vi "Triaxial Aquisition.vi"() -> ()   [LabVIEW 2017]
uses:
  <vilib>/UPVI/lvhdf5/dataset.llb/LVH5D Operation.ctl
  <vilib>/Utility/miscctls.llb/LVRectTypeDef.ctl
  <vilib>/UPVI/lvhdf5/attribute.llb/LVH5A Operation.ctl
  <vilib>/UPVI/lvhdf5/group.llb/H5G_obj_t.ctl
  <vilib>/UPVI/lvhdf5/file.llb/LVH5F Operation.ctl
  <vilib>/UPVI/lvhdf5/identifier.llb/Not an HDF5 Refnum Constant.vi
  <vilib>/UPVI/lvhdf5/common.llb/To HDF5 Ref.vi
  <vilib>/express/express analysis/Spectral/Block/exnSpectralBlock spectral measurements power poly.vi
  <vilib>/express/express analysis/Spectral/Block/exnSpectralBlock spectral measurements power DDT.vi
  <vilib>/UPVI/lvhdf5/file.llb/OpenCreateReplace HDF5 File.vi
  <vilib>/UPVI/lvhdf5/utility.llb/Select HDF5 Dialog.vi
  <vilib>/UPVI/lvhdf5/utility.llb/Select HDF5 Dialog (File and Object).vi
  <vilib>/UPVI/lvhdf5/dataset.llb/Simple H5Dwrite (Variant).vi
  <vilib>/UPVI/lvhdf5/attribute.llb/Write Multiple Attributes.vi
  <vilib>/UPVI/lvhdf5/dataset.llb/H5Dclose.vi
  <vilib>/express/express analysis/Spectral/XNode/ExpressSpectralMeasurementsBlockNode.xnode
  <vilib>/UPVI/lvhdf5/dataset.llb/Write Dataset with Attributes.xnode
  <vilib>/UPVI/lvhdf5/library.llb/HDF5 Ref.ctl
  <vilib>/Utility/error.llb/Error Cluster From Error Code.vi
  <vilib>/UPVI/lvhdf5/dataset.llb/OpenCreateReplace Dataset by Element Type.vi
  <vilib>/UPVI/lvhdf5/dataspace.llb/H5Sselect_hyperslab.vi
  <vilib>/UPVI/lvhdf5/dataset.llb/H5Dwrite (Variant).vi
  <vilib>/UPVI/lvhdf5/dataset.llb/H5Dget_space.vi
  <vilib>/UPVI/lvhdf5/attribute.llb/private/LVH5AwriteWDTAttrs.vi
  <vilib>/UPVI/lvhdf5/dataspace.llb/H5Sclose.vi
  <vilib>/UPVI/lvhdf5/utility.llb/Select HDF5 Dialog (Object Only).vi
  <vilib>/Utility/VariantDataType/GetClusterInfo.vi
  <vilib>/Utility/VariantDataType/VariantType.lvlib
  <vilib>/Utility/VariantDataType/GetTypeInfo.vi
  <vilib>/UPVI/lvhdf5/attribute.llb/Cluster to Attribute Array.xnode
panel:
  out "Array":dbl[][](array[numeric])
  out "Z":dynamicdata(graph)
  out "Y":dynamicdata(graph)
  out "X":dynamicdata(graph)
  out "data 3":dynamicdata(graph) caption="Z"
  out "data 2":dynamicdata(graph) caption="Y"
  out "data":dynamicdata(graph) caption="X"
  in  "stop (F)":bool
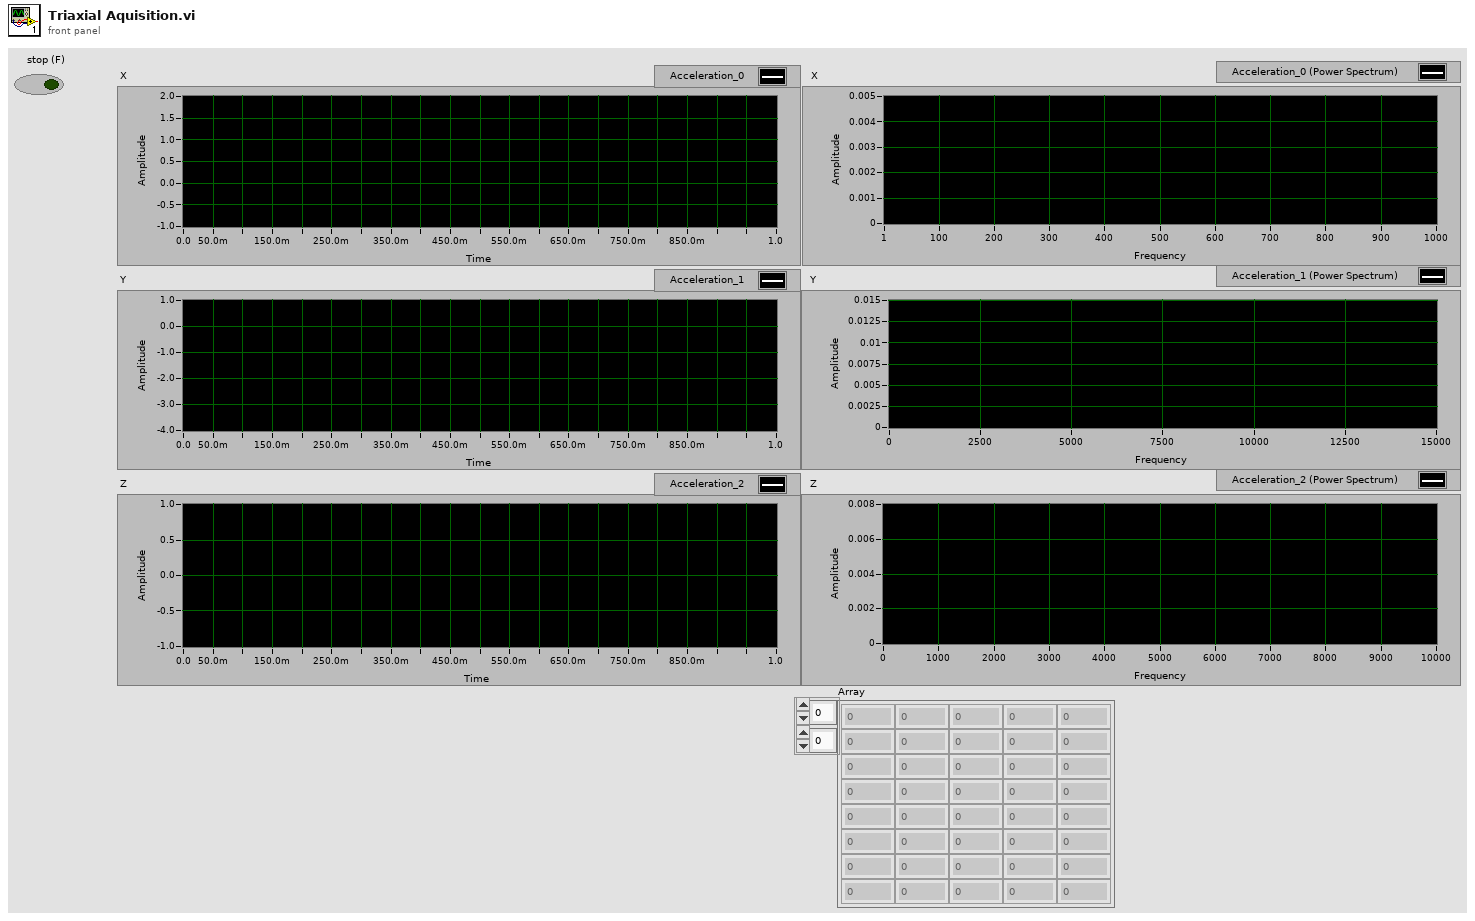
[diagram p1: front panel]
types:
  T1 = typedef "LVH5D Operation.ctl" = enum16{"open", "replace", "create", "open or create", "create or replace", "create or replace with confirmation"}
  T2 = typedef "HDF5 Ref.ctl" = refnum<k1>
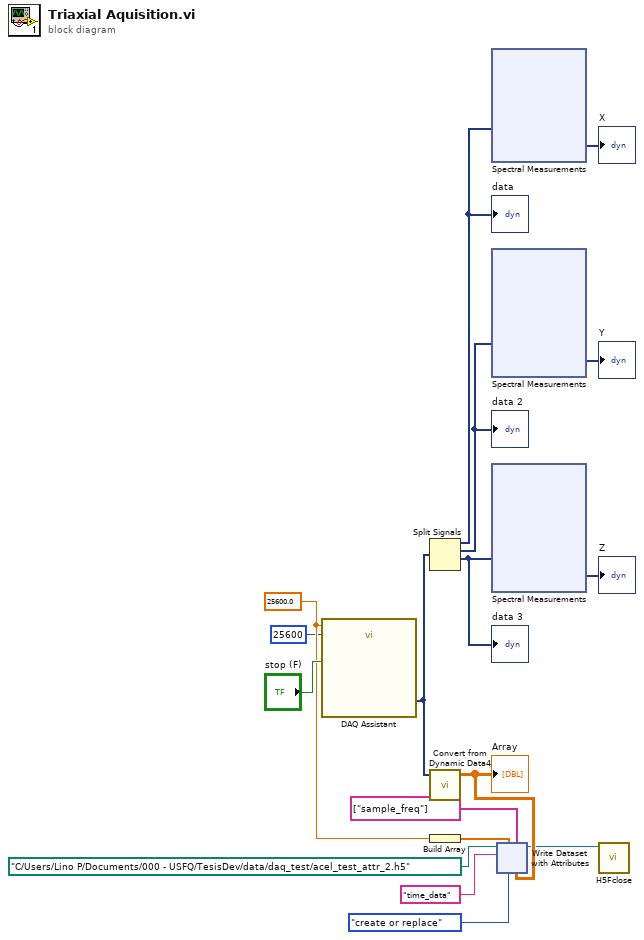
[diagram p0: block diagram]
diagram:
  w3 = 25600.0 ("rate")
  n1 = call "DAQ Assistant"("rate"=w3, "number of samples"=25600, "stop (T)"="stop (F)") -> ("data"=w10:dynamicdata)  [unwired: 14 in, 2 out]
  n2 = Split Signals(w10) -> (w13:dynamicdata, w15:dynamicdata, w11:dynamicdata)  [unwired: 4 in, 1 out]
  "data" <- w13
  "data 2" <- w15
  "data 3" <- w11
  n3 = call "Convert from Dynamic Data4"("Dynamic Data Type"=w10) -> ("Array"=w9:dbl[][])  [unwired: 3 in]
  "Array" <- w9
  n4 = Build Array(w3) -> (w2:dbl[])
  n5 = xnode "Spectral Measurements"("Signals"=w13) -> ("Power Spectrum"=→"X":dynamicdata)  [unwired: 1 in, 1 out]
  n6 = xnode "Spectral Measurements"("Signals"=w15) -> ("Power Spectrum"=→"Y":dynamicdata)  [unwired: 1 in, 1 out]
  n7 = xnode "Spectral Measurements"("Signals"=w11) -> ("Power Spectrum"=→"Z":dynamicdata)  [unwired: 1 in, 1 out]
  n8 = xnode "Write Dataset with Attributes"("Dataset Path"="time_data", "operation (open or create)"=LVH5D_Operation."create or replace", "HDF5 Path or Ref"=path "C:/Users/Lino P/Documents/000 - USFQ/TesisDev/data/daq_test/acel_test_attr_2.h5" ("path"), "Attribute Name(s)"=string[] ["sample_freq"], "Attribute Value(s)"=w2, "Data"=w9) -> ("HDF5 Ref out"=w5:T2)  [unwired: 2 in, 2 out]
  n9 = call <vilib>:"H5Fclose.vi"("HDF5 Ref"=w5) -> ()  [unwired: 8 in, 1 out]
